vi "Ejercicio 3.2.vi"() -> ()   [LabVIEW 2021]
panel:
  out "Subcadena situado el lugar 20 y 30:":string
  out "Longitud Total de cadena:":string
  out "Vocal más repetida:":string
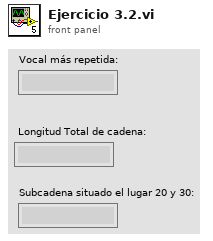
[diagram p1: front panel]
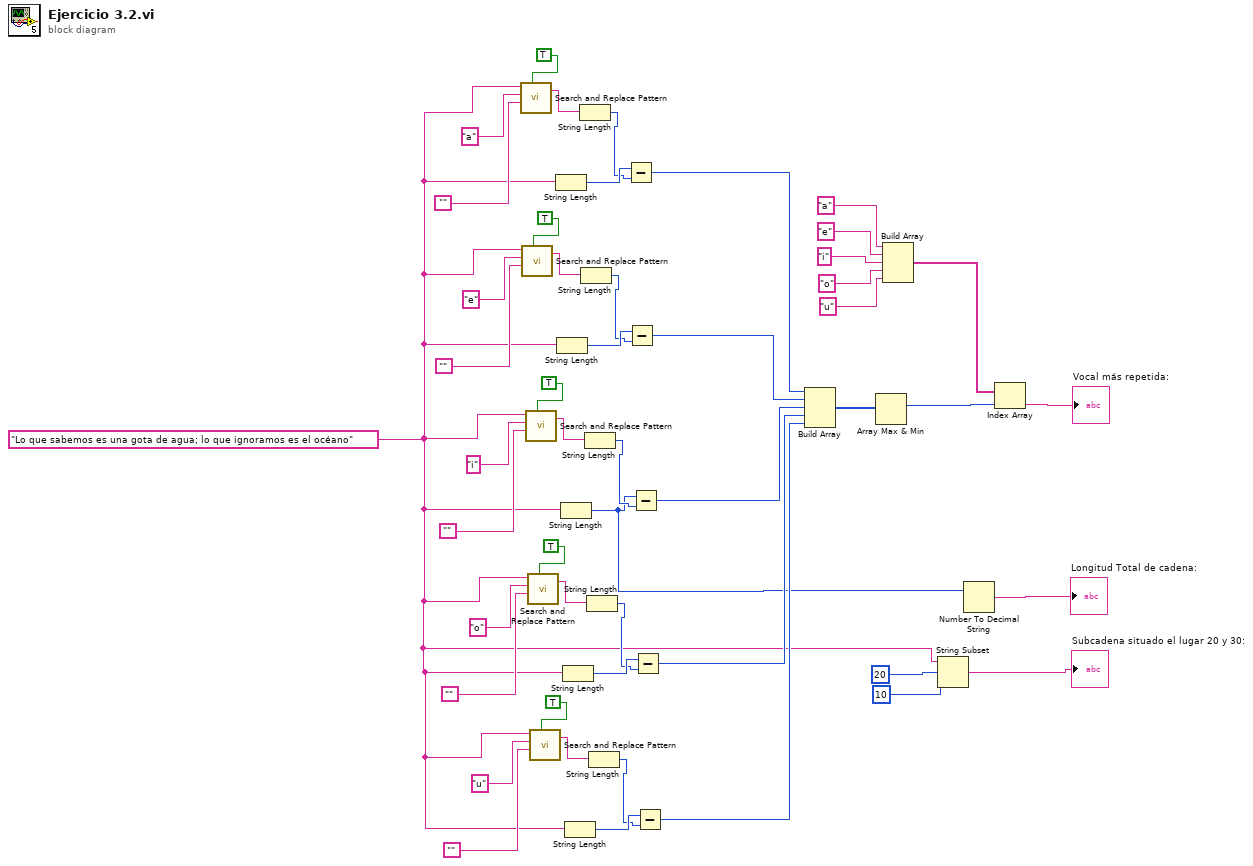
[diagram p0: block diagram]
diagram:
  w4 = "Lo que sabemos es una gota de agua; lo que ignoramos es el océano"
  n1 = call <vilib>:"Search and Replace Pattern.vi"("string"=w4, "regular expression (\"\")"="a", "replace string (\"\")"="", "replace all? (F)"=TRUE) -> ("result string"=w8:string)  [unwired: 1 in, 1 out]
  n2 = call <vilib>:"Search and Replace Pattern.vi"("string"=w4, "regular expression (\"\")"="e", "replace string (\"\")"="", "replace all? (F)"=TRUE) -> ("result string"=w41:string)  [unwired: 1 in, 1 out]
  n3 = call <vilib>:"Search and Replace Pattern.vi"("string"=w4, "regular expression (\"\")"="i", "replace string (\"\")"="", "replace all? (F)"=TRUE) -> ("result string"=w35:string)  [unwired: 1 in, 1 out]
  n4 = call <vilib>:"Search and Replace Pattern.vi"("string"=w4, "regular expression (\"\")"="o", "replace string (\"\")"="", "replace all? (F)"=TRUE) -> ("result string"=w30:string)  [unwired: 1 in, 1 out]
  n5 = call <vilib>:"Search and Replace Pattern.vi"("string"=w4, "regular expression (\"\")"="u", "replace string (\"\")"="", "replace all? (F)"=TRUE) -> ("result string"=w24:string)  [unwired: 1 in, 1 out]
  n6 = String Length(string=w4) -> (length=w46:i32)
  n7 = String Length(string=w4) -> (length=w40:i32)
  n8 = String Length(string=w4) -> (length=w7:i32)
  n9 = String Length(string=w4) -> (length=w29:i32)
  n10 = String Length(string=w4) -> (length=w23:i32)
  n11 = String Length(string=w8) -> (length=w45:i32)
  n12 = String Length(string=w41) -> (length=w39:i32)
  n13 = String Length(string=w35) -> (length=w34:i32)
  n14 = String Length(string=w30) -> (length=w28:i32)
  n15 = String Length(string=w24) -> (length=w22:i32)
  n16 = Subtract(x=w46, y=w45) -> (x-y=w21:i32)
  n17 = Subtract(x=w40, y=w39) -> (x-y=w20:i32)
  n18 = Subtract(x=w7, y=w34) -> (x-y=w19:i32)
  n19 = Subtract(x=w29, y=w28) -> (x-y=w18:i32)
  n20 = Subtract(x=w23, y=w22) -> (x-y=w17:i32)
  n21 = Build Array(w21, w20, w19, w18, w17) -> (w16:i32[])
  n22 = Array Max & Min(array=w16) -> (max index (indices)=w9:i32)  [unwired: 3 out]
  n23 = Build Array("a", "e", "i", "o", "u") -> (w10:string[])
  n24 = String Subset(string=w4, offset (0)=20, length (rest)=10) -> (substring=→"Subcadena situado el lugar 20 y 30:":string)
  n25 = Number To Decimal String(number=w7) -> (decimal integer string=→"Longitud Total de cadena:":string)  [unwired: 1 in]
  n26 = Index Array(array=w10, index=w9) -> (element=→"Vocal más repetida:":string)
